vi "Write Binary Config.vi"(4 "Include Class Name":bool, 6 "byte order (0:big-endian, network order)":T1(ring), 8 "error in (no error)":errorcluster, 11 "abs_SharedVar_Bool in":refnum<class "conc_SharedVar_I16.lvclass">) -> (0 "error out":errorcluster, 2 "Binary":string, 3 "abs_SharedVar_Bool out":refnum<class "conc_SharedVar_I16.lvclass">)   [LabVIEW 2021, in "conc_SharedVar_I16.lvclass"]
uses:
  conc_SharedVar_I16.lvclass
  conc_SharedVar_I16.lvclass/conc_SharedVar_I16.ctl
  <vilib>/TSA/Abstract Data Classes/Abs_Types/I16 Integer/Abs_I16 Integer.lvclass
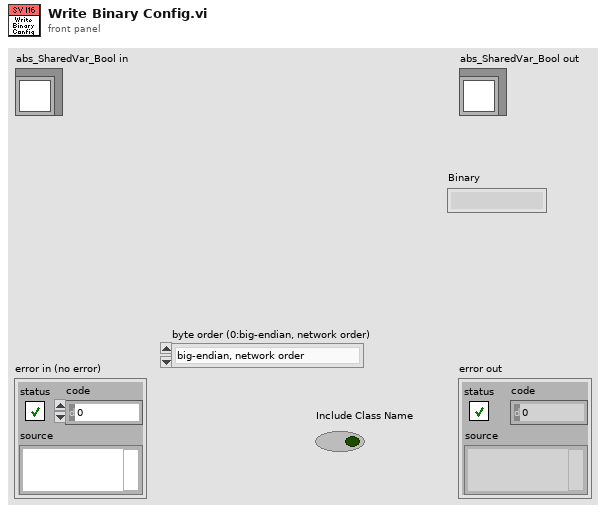
[diagram p1: front panel]
types:
  T1 = enum16{"big-endian, network order", "native, host order", "little-endian"}
  T2 = cluster{"Shared Variable Refnum":refnum<k21>, "Write Access":enum8{"Allowed", "Required", "None"}, "Read Access":enum8{"Allowed", "Required", "None"}}
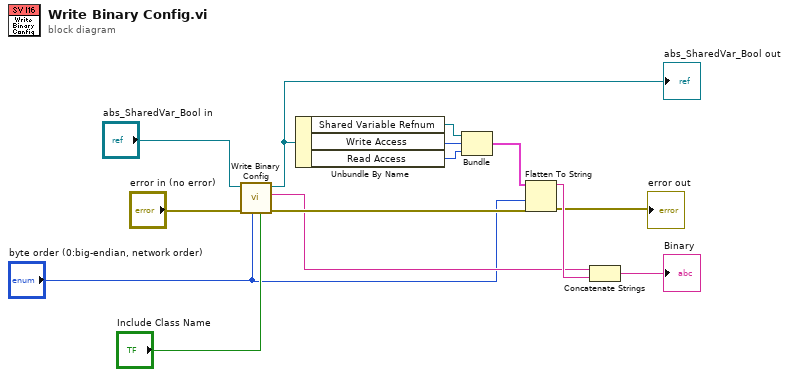
[diagram p0: block diagram]
diagram:
  n1 = call-parent "Write Binary Config.vi"("Include Class Name"="Include Class Name", "byte order (0:big-endian, network order)"="byte order (0:big-endian, network order)", "error in (no error)"="error in (no error)", "Abs_Type in"="abs_SharedVar_Bool in") -> ("error out"=w10:errorcluster, "Binary"=w9:string, "Abs_Type out"=w7:refnum<class "conc_SharedVar_I16.lvclass">)  [unwired: 5 in]
  "abs_SharedVar_Bool out" <- w7
  n2 = Unbundle By Name(w7) -> ("Shared Variable Refnum"=w6:refnum<k21>, "Write Access"=w5:enum8{"Allowed", "Required", "None"}, "Read Access"=w4:enum8{"Allowed", "Required", "None"})
  n3 = Bundle("Shared Variable Refnum"=w6, "Write Access"=w5, "Read Access"=w4) -> (w3:T2)  [unwired: 1 in]
  n4 = Flatten To String(anything=w3, byte order (0:big-endian, network order)="byte order (0:big-endian, network order)", error in (no error)=w10) -> (data string=w11:string, error out=→"error out":errorcluster)  [unwired: 1 in, 1 out]
  n5 = Concatenate Strings(w9, w11) -> (→"Binary":string)
